vi "Exemple_Preprocessing_robust_scale.vi"() -> ()   [LabVIEW 2020]
panel:
  out "Data":T1
  out "error out":errorcluster
  in  "X":string[][](array[string])=[["1", "-2", "2"], ["-2", "1", "3"], ["4", "1", "-2"]]
  in  "error in":errorcluster caption="entrée d'erreur"
  in  "robust_scale":T2={"axis"=0, "with_centering"=TRUE, "with_scaling"=TRUE, "quantile_range"={"q_min"=25.0, "q_max"=75.0}, "copy"=TRUE}
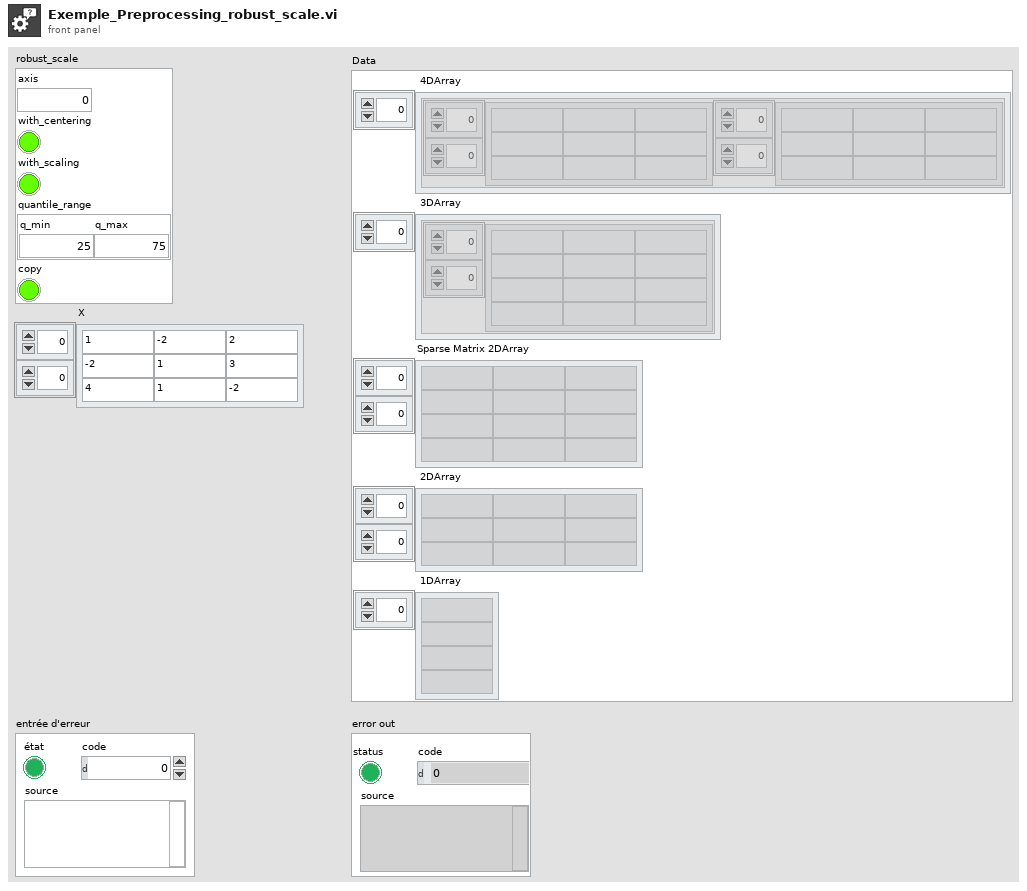
[diagram p1: front panel]
types:
  T1 = cluster{" 4DArray":cluster{"1":string[][], "2":string[][]}[], " 3DArray":cluster{"Tableau":string[][]}[], "Sparse Matrix 2DArray":string[][], " 2DArray":string[][], " 1DArray":string[]}
  T2 = cluster{"axis":i32, "with_centering":bool, "with_scaling":bool, "quantile_range":cluster{"q_min":dbl, "q_max":dbl}, "copy":bool}
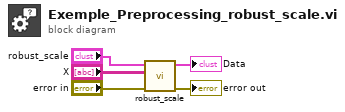
[diagram p0: block diagram]
diagram:
  n1 = call "robust_scale.vi"("error in"="error in", "X"="X", "robust_scale"="robust_scale") -> ("error out"=→"error out":errorcluster, "Data"=→"Data":T1)  [unwired: 7 in]
